vi "AverageTIFFs.vi"(0 "file path":path=path "\\\\BIZ-SERVER\\Messdaten/Entwicklung/SI/20130308-1080wobtest/8160_cropcombine.tif") -> ()   [LabVIEW 2011]
uses:
  TiffModules/AddTiffPage_U16_text_res.vi
panel:
  out "s? t:f":enum16{"first", "mid", "last"}(ring)
  in  "Frames to average; 0=all":i32=7
  out "Input-page":i32=156
  out "string":string
  out "xy-resolution":cluster{"x":dbl, "y":dbl}
  out "Out":u16[][](graph)
  out "In":u16[][](graph)
  # "select a tiff file,\nEnter average Number\nrun\nappended tif with name_average#.tif"
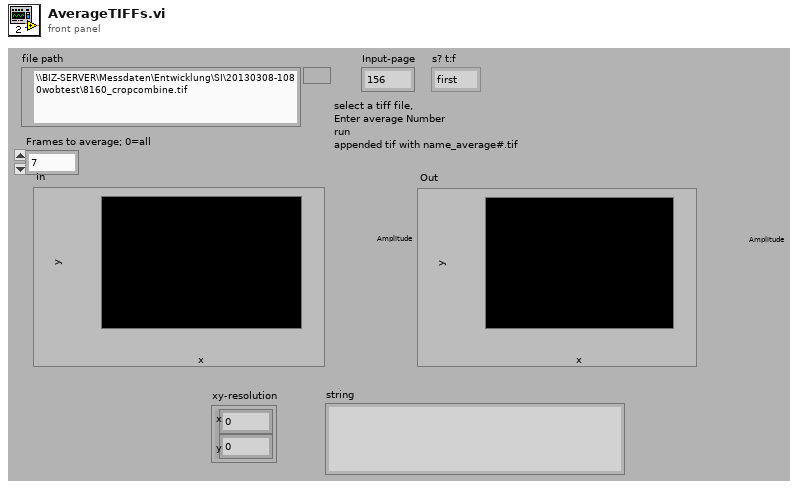
[diagram p1: front panel]
types:
  T1 = cluster{"Tiff refnum":refnum<file>, "Byte-Reihenfolge (0:Big-Endian, 2:LSB)":enum16{"big-endian, network order", "native, host order", "little-endian"}}
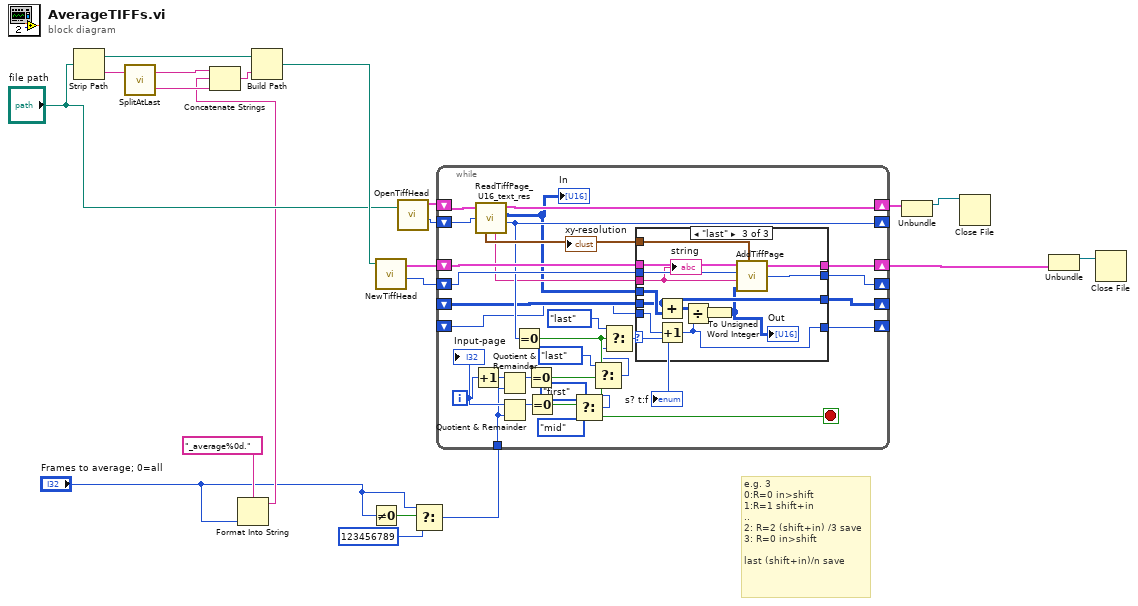
[diagram p0: block diagram]
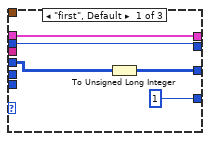
[diagram p2: hidden frame]
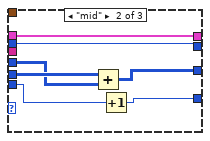
[diagram p3: hidden frame]
diagram:
  # "e.g. 3\n0:R=0 in>shift\n1:R=1 shift+in\n..\n2: R=2 (shift+in) /3 save\n3: R=0 in>shift\n\nlast (shift+in)/n save"
  n1 = Strip Path(path="file path") -> (stripped path=w12:path, name=w13:string)
  n2 = call "SplitAtLast.vi"("In-String"=w13) -> ("end"=w21:string, "Front (default)"=w14:string)  [unwired: 1 in]
  n3 = Format Into String(format string="_average%0d.", "Frames to average; 0=all") -> (resulting string=w5:string)  [unwired: 2 in, 1 out]
  n4 = Concatenate Strings(w14, w5, w21) -> (w20:string)
  n5 = Build Path(base path=w12, name or relative path=w20) -> (appended path=w19:path)
  n6 = Not Equal To 0?(x="Frames to average; 0=all") -> (x != 0?=w4:bool)
  n7 = call "NewTiffHead.vi"("file path"=w19) -> ("TIFF file"=w18:T1, "Place for first IFD (8,eof-position)"=w17:u32)  [unwired: 3 in, 1 out]
  n8 = call "OpenTiffHead.vi"("file path"="file path") -> ("TIFF file"=w11:T1, "first Diroffset"=w10:u32)  [unwired: 2 in, 1 out]
  n9 = Select(t="Frames to average; 0=all", s=w4, f=123456789) -> (s? t:f=w2:i32)
  n10 = while {
    shift-right: [w45] -> w9
    shift-left: w11 -> [w48]
    shift-right: [w50] -> w16
    shift-left: w18 -> [w51]
    shift-right: [w44] -> _
    shift-left: w10 -> [w47]
    shift-right: [w42] -> _
    shift-left: w17 -> [w49]
    shift-right: [w40] -> _
    shift-left: _ -> [w39]
    tunnel: w2 -> [w36]
    shift-right: [w23] -> _
    shift-left: _ -> [w22]
    i -> [w37]
    stop <- w33 stop-if-true
    n11 = Increment(x=w37) -> (x+1=w38:i32)
    n12 = call "ReadTiffPage_U16_text_res.vi"("TIFF file"=w48, "IFDoffset"=w47) -> ("Pixelsize [µm]"=w46:cluster{"x":dbl, "y":dbl}, "TIFF file out"=w45:T1, "16-bit pixmap"=w41:u16[][], "string"=w43:string, "Next offset"=w44:i32)  [unwired: 3 in, 1 out]
    "In" <- w41
    "xy-resolution" <- w46
    n13 = Quotient & Remainder(x=w38, y=w36) -> (x-y*floor(x/y)=w35:i32)  [unwired: 1 out]
    n14 = Quotient & Remainder(x=w37, y=w36) -> (x-y*floor(x/y)=w34:i32)  [unwired: 1 out]
    n15 = Equal To 0?(x=w44) -> (x = 0?=w33:bool)
    n16 = Equal To 0?(x=w35) -> (x = 0?=w26:bool)
    n17 = Equal To 0?(x=w34) -> (x = 0?=w30:bool)
    n18 = Select(t=enum16{"first", "mid", "last"}."first", s=w30, f=enum16{"first", "mid", "last"}."mid") -> (s? t:f=w25:enum16{"first", "mid", "last"})
    n19 = Select(t=enum16{"first", "mid", "last"}."last", s=w26, f=w25) -> (s? t:f=w24:enum16{"first", "mid", "last"})
    n20 = Select(t=enum16{"first", "mid", "last"}."last", s=w33, f=w24) -> (s? t:f=w31:enum16{"first", "mid", "last"})
    "s? t:f" <- w31
    n21 = case shown="\"last\"" w31 {
      tunnel: w51 -> [w56 w63 w76]
      tunnel: [w56 w63 w75] -> w50
      tunnel: w49 -> [w55 w62 w71]
      tunnel: w46 -> [_ _ w74]
      tunnel: w43 -> [_ _ w68]
      tunnel: [w55 w62 w73] -> w42
      tunnel: w41 -> [w54 w59 w70]
      tunnel: [w53 w61 w67] -> w40
      tunnel: w39 -> [_ w60 w67]
      tunnel: [1 w58 w64] -> w23
      tunnel: w22 -> [_ w57 w65]
      frame "first", Default {
        n22 = To Unsigned Long Integer(number=w54) -> (unsigned 32bit integer=w53:u32[][])
      }
      frame "mid" {
        n23 = Add(x=w60, y=w59) -> (x+y=w61:u32[][])
        n24 = Increment(x=w57) -> (x+1=w58:i32)
      }
      frame "last" {
        n25 = Add(x=w67, y=w70) -> (x+y=w69:u32[][])
        n26 = Increment(x=w65) -> (x+1=w64:i32)
        n27 = Divide(x=w69, y=w64) -> (x/y=w72:dbl[][])
        n28 = To Unsigned Word Integer(number=w72) -> (unsigned 16bit integer=w66:u16[][])
        "Out" <- w66
        n29 = call-poly "AddTiffPage.vi"("TIFF file"=w76, "After last DIROffset"=w71, "Text"=w68, "16-bit pixmap x, y"=w66, "Pixelsize [µm]"=w74) -> ("TIFF file out"=w75:T1, "AfterDIRoffset"=w73:u32)  [unwired: 1 out]
        "string" <- w68
      }
    }
    "Input-page" <- w37
  }
  n30 = Unbundle(w9) -> ("Tiff refnum"=w8:refnum<file>)  [unwired: 1 out]
  n31 = Close File(refnum=w8) -> ()  [unwired: 1 in, 2 out]
  n32 = Unbundle(w16) -> ("Tiff refnum"=w15:refnum<file>)  [unwired: 1 out]
  n33 = Close File(refnum=w15) -> ()  [unwired: 1 in, 2 out]
